vi "check_and_correct_input.vi"() -> ()   [LabVIEW 2011]
panel:
  in  "delay array 2":dbl[](array[numeric])
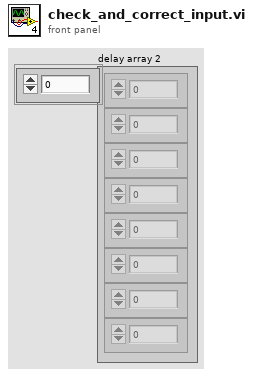
[diagram p1: front panel]
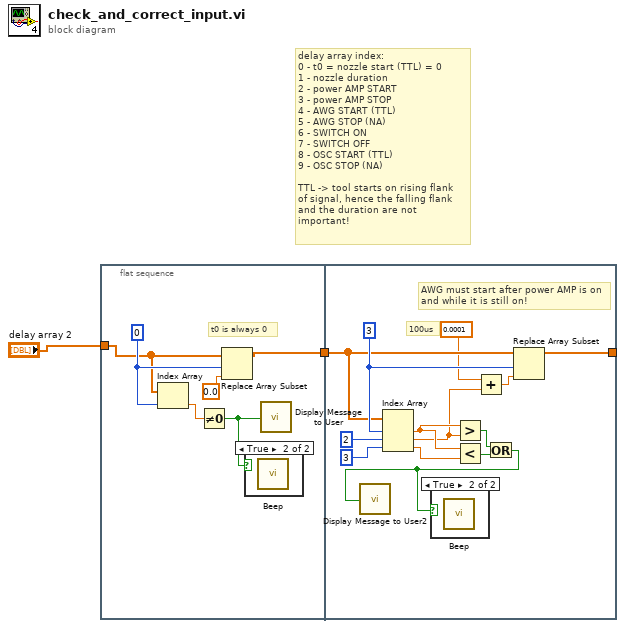
[diagram p0: block diagram]
diagram:
  # "delay array index:\n0 - t0 = nozzle start (TTL) = 0\n1 - nozzle duration\n2 - power AMP START\n3 - power AMP STOP\n4 - AWG START (TTL)\n5 - AWG STOP (NA)\n6 - SWITCH ON \n7 - SWITCH OFF\n8 - OSC START (TTL)\n9 - OSC STOP (NA)\n\nTTL -> tool starts on rising flank\nof signal, hence the falling flank \nand the duration are not important!"
  n1 = flat-sequence {
    tunnel: "delay array 2" -> [w5]
    tunnel: [w4] -> w1
    tunnel: [w21] -> _
    tunnel: w1 -> [w17]
    frame #0 {
      w6 = 0 ("index")
      # "t0 is always 0"
      n2 = Index Array(array=w5, index=w6) -> (element=w7:dbl)
      n3 = Not Equal To 0?(x=w7) -> (x != 0?=w3:bool)
      n4 = Replace Array Subset(array=w5, new element=0.0 ("new element/subarray"), index=w6) -> (w4:dbl[])
      n5 = case shown="True" w3 {
        frame False {
        }
        frame True {
          n6 = call <vilib>:"Beep.vi"() -> ()  [unwired: 12 in]
        }
      }
      n7 = call "Display Message to User"("Enable"=w3) -> ()  [unwired: 9 in, 2 out]
    }
    frame #1 {
      w20 = 3 ("index")
      # "100us"
      # "AWG must start after power AMP is on \nand while it is still on!"
      n8 = Index Array(array=w17, index #1=w20, index #2=2 ("index"), index #3=3 ("index")) -> (element #1=w15:dbl, element #2=w11:dbl, element #3=w14:dbl)
      n9 = Greater?(x=w15, y=w11) -> (0:w16:bool)
      n10 = Less?(x=w15, y=w14) -> (x < y?=w13:bool)
      n11 = Add(x=0.0001, y=w11) -> (x+y=w9:dbl)
      n12 = Or(x=w16, y=w13) -> (x .or. y?=w10:bool)
      n13 = call "Display Message to User2"("Enable"=w10) -> ()  [unwired: 9 in, 2 out]
      n14 = case shown="True" w10 {
        frame False {
        }
        frame True {
          n15 = call <vilib>:"Beep.vi"() -> ()  [unwired: 12 in]
        }
      }
      n16 = Replace Array Subset(array=w17, new element=w9, index=w20) -> (w21:dbl[])
    }
  }
